vi "calcMirRotMat.vi"(8 "error in (no error)":errorcluster, 10 "Rotation Angle in Deg":dbl, 11 "CamRot in":refnum<class "CamRot.lvclass">) -> (0 "error out":errorcluster, 2 "Rotation Matrix":dbl[][](array[numeric]), 3 "CamRot out":refnum<class "CamRot.lvclass">)   [LabVIEW 2016, in "CamRot.lvclass"]
doc: "Calculate the mirror rotation matrix."
uses:
  CamRot.lvclass
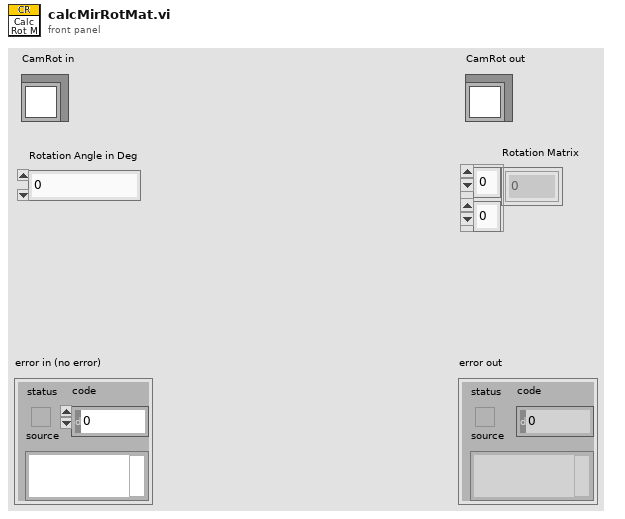
[diagram p1: front panel]
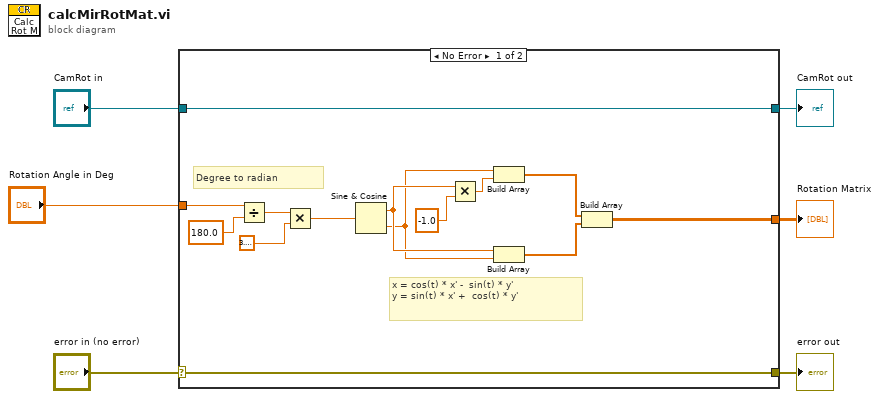
[diagram p0: block diagram]
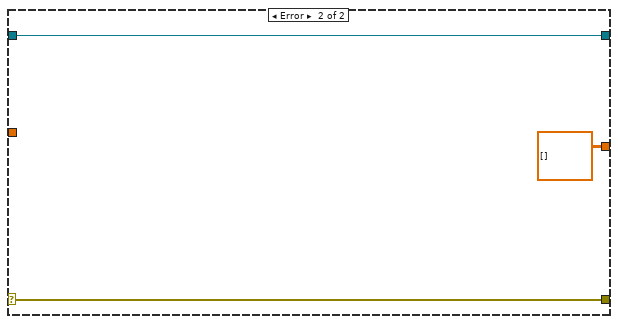
[diagram p2: hidden frame]
diagram:
  n1 = case shown="No Error" "error in (no error)" {
    selector: "error in (no error)" -> [w19 w23]
    tunnel: [w19 w23] -> w5
    tunnel: [w20 w22] -> w3
    tunnel: "CamRot in" -> [w20 w22]
    tunnel: "Rotation Angle in Deg" -> [w18 _]
    tunnel: [w7 dbl[][] []] -> w1
    frame No Error {
      # "x = cos(t) * x' -  sin(t) * y'\ny = sin(t) * x' +  cos(t) * y'"
      # "Degree to radian"
      n2 = Divide(x=w18, y=180.0) -> (x/y=w16:dbl)
      n3 = Multiply(x=w16, y=3.141592653589793) -> (x*y=w14:dbl)
      n4 = Sine & Cosine(0:w14) -> (1:w11:dbl, 2:w10:dbl)
      n5 = Multiply(x=w11, y=-1.0) -> (x*y=w12:dbl)
      n6 = Build Array(w10, w12) -> (w9:dbl[])
      n7 = Build Array(w11, w10) -> (w8:dbl[])
      n8 = Build Array(w9, w8) -> (w7:dbl[][])
    }
    frame Error {
    }
  }
  "error out" <- w5
  "CamRot out" <- w3
  "Rotation Matrix" <- w1
